vi "Transform E1, E2 using map calib xform_PN.vi"(2 "Sx, Tx, Sy, Ty":dbl[](array[numeric])=[1.0000263372329348, -5.817138285027323e-05, 0.9999727510054321, 6.062261811624134e-05], 3 "S*cos(q), S*sin(q), Tx, Ty":dbl[](array[numeric])=[1.0763223002323654, 0.0007524070719776288, -0.14779165640104555, -0.09827403757225917], 4 "E2/G2 + O2 orig":dbl[](array[numeric])=[1.8385477776704264, 1.9097301929305215, 2.0217441886705823, 2.102764185952928, 2.1689565980547436, 2.223597346902293, 2.313108622344049, 2.386560175928841, 2.4493106687615236, 2.5040748520274185, 2.5540239094260055], 5 "E1/G1 + O1 orig":dbl[](array[numeric])=[1.8159023665858196, 1.884909478785341, 2.0019297168656713, 2.086321368481948, 2.153544842540943, 2.2091798744386204, 2.299969711011518, 2.3739532300327273, 2.436788143576289, 2.4919329317716272, 2.5414088647043536]) -> (0 "E2/G2 + O2 xformed":dbl[](array[numeric])=[1.8819715743991605, 1.958636627664691, 2.0792845484484253, 2.1665492972222093, 2.2378423031751806, 2.2966936161698364, 2.3931022818543477, 2.472213336931841, 2.539798527472872, 2.598782323211661, 2.65257936765186], 1 "E1/G1 + O1 xformed":dbl[](array[numeric])=[1.8053105952325403, 1.8795328855731468, 2.005403412269025, 2.0961774595124005, 2.1684836843979456, 2.22832537384071, 2.3259797225395, 2.4055566642245805, 2.473141848949985, 2.5324557713908873, 2.585671640828993])   [LabVIEW 2010]
uses:
  <vilib>/Analysis/Matrix/Numeric/Conversions/Array To Matrix - RA2.vi
  <vilib>/Analysis/baseanly.llb/A x Vector.vi
  <vilib>/Analysis/Matrix/NI_Matrix.lvlib
  <vilib>/Analysis/NI_AALBase.lvlib
panel:
  out "E1, E2 corrected and un-corrected against calib.":cluster{dbl[], dbl[]}[](graph)=[{[1.8159023665858196, 1.884909478785341, 2.0019297168656713, 2.086321368481948, 2.153544842540943, 2.2091798744386204, 2.299969711011518, 2.3739532300327273, 2.436788143576289, 2.4919329317716272, 2.5414088647043536], [1.8385477776704264, 1.9097301929305215, 2.0217441886705823, 2.102764185952928, 2.1689565980547436, 2.223597346902293, 2.313108622344049, 2.386560175928841, 2.4493106687615236, 2.5040748520274185, 2.5540239094260055]}, {[1.8053105952325403, 1.8795328855731468, 2.005403412269025, 2.0961774595124005, 2.1684836843979456, 2.22832537384071, 2.3259797225395, 2.4055566642245805, 2.473141848949985, 2.5324557713908873, 2.585671640828993], [1.8819715743991605, 1.958636627664691, 2.0792845484484253, 2.1665492972222093, 2.2378423031751806, 2.2966936161698364, 2.3931022818543477, 2.472213336931841, 2.539798527472872, 2.598782323211661, 2.65257936765186]}]
  # "Paul Nathan 16/02/10"
  # "Transformation equations given below"
  # "First apply uniform scaling with rotation and translation:"
  # "then apply independent scaling with translation onto the points mapped with the above transformation (as a final correction, typically small)"
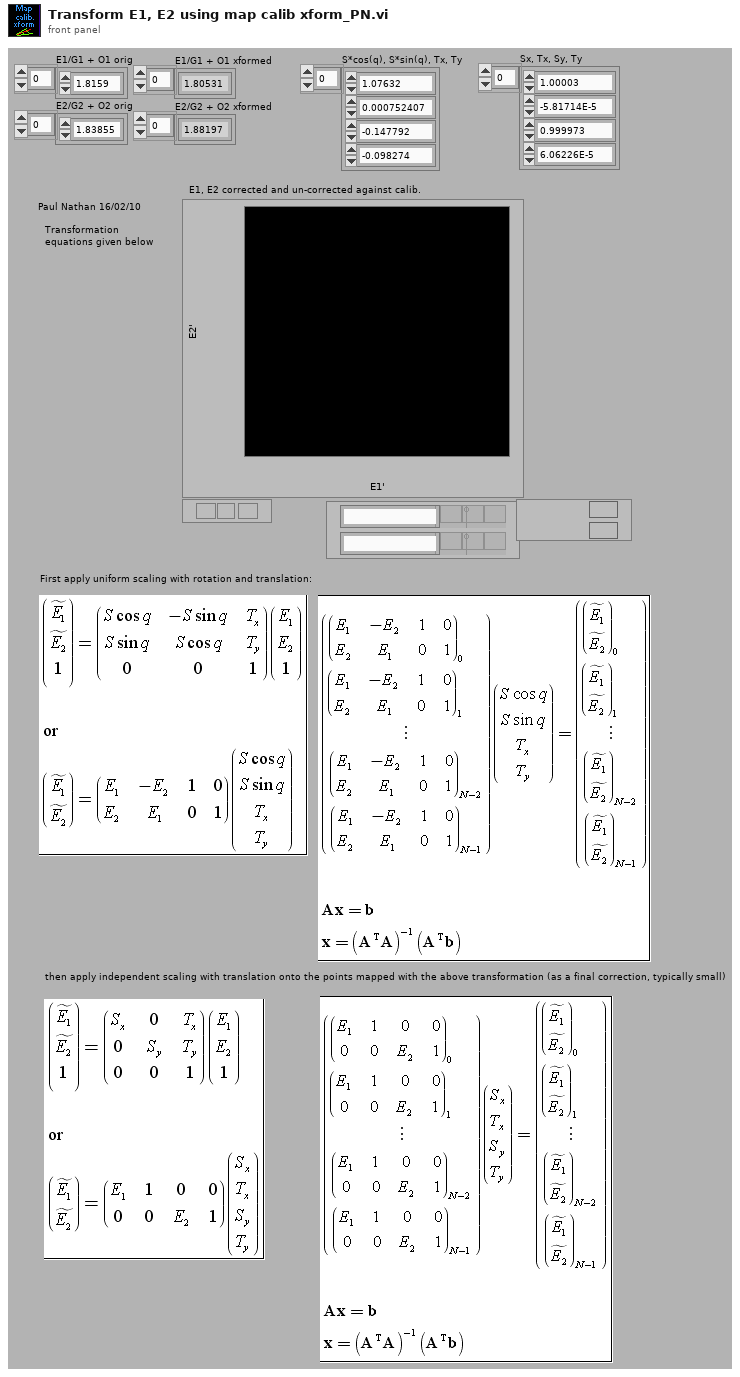
[diagram p1: front panel]
types:
  T1 = cluster{"E1/G1 + O1 orig":dbl[], "E2/G2 + O2 orig":dbl[]}
  T2 = typedef "NI_Matrix.lvlib/RealMatrix.ctl" = dbl[][]
  T3 = cluster{"E1/G1 + O1 orig":dbl[], "E2/G2 + O2 orig":dbl[]}[]
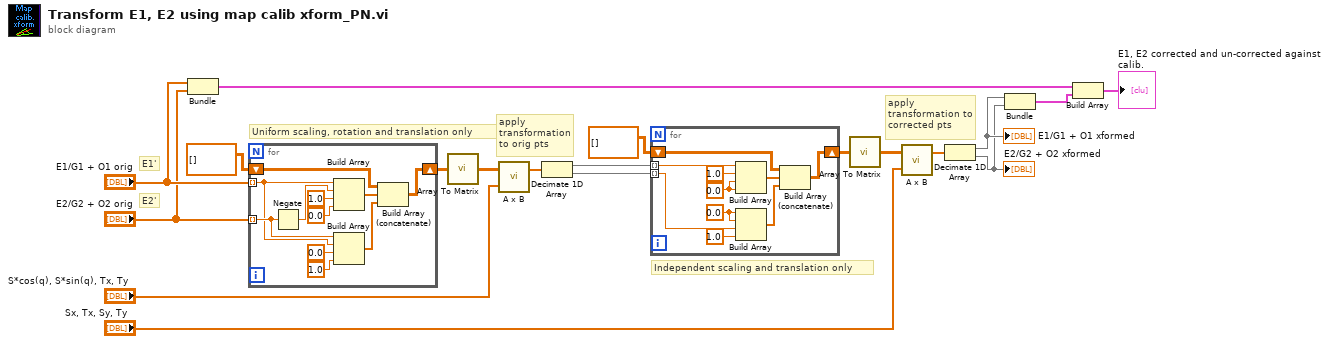
[diagram p0: block diagram]
diagram:
  # "apply transformation to corrected pts"
  # "apply transformation to orig pts"
  # "Independent scaling and translation only"
  # "Uniform scaling, rotation and translation only"
  # "E2'"
  # "E1'"
  n1 = Bundle("E1/G1 + O1 orig"="E1/G1 + O1 orig", "E2/G2 + O2 orig"="E2/G2 + O2 orig") -> (w6:T1)  [unwired: 1 out]
  n2 = for {
    tunnel: "E1/G1 + O1 orig" -> [w24] mode=indexing
    tunnel: "E2/G2 + O2 orig" -> [w25] mode=indexing
    shift-right: [w23] -> w16
    shift-left: dbl[][] [] -> [w22]
    n3 = Negate(x=w25) -> (-x=w30:dbl)
    n4 = Build Array(w24, w30, 1.0 ("element"), 0.0 ("element")) -> (w21:dbl[])
    n5 = Build Array(w25, w24, 0.0 ("element"), 1.0 ("element")) -> (w20:dbl[])
    n6 = Build Array (concatenate)(w22, w21, w20) -> (w23:dbl[][])
  }
  n7 = call-poly <vilib>:"Array To Matrix.vi"("Real 2D Array"=w16) -> ("Real Matrix"=w15:T2)
  n8 = call-poly <vilib>:"A x B.vi"("Vector"="S*cos(q), S*sin(q), Tx, Ty", "A"=w15) -> ("A x Vector"=w14:dbl[])  [unwired: 1 out]
  n9 = Decimate 1D Array(w14) -> (w12:dbl[], w13:dbl[])
  n10 = for {
    tunnel: w12 -> [w39] mode=indexing
    tunnel: w13 -> [w33] mode=indexing
    shift-right: [w38] -> w18
    shift-left: dbl[][] [] -> [w37]
    w31 = 0.0 ("element")
    w32 = 0.0 ("element")
    n11 = Build Array(w39, 1.0 ("element"), w32, w32) -> (w36:dbl[])
    n12 = Build Array(w31, w31, w33, 1.0 ("element")) -> (w35:dbl[])
    n13 = Build Array (concatenate)(w37, w36, w35) -> (w38:dbl[][])
  }
  n14 = call-poly <vilib>:"Array To Matrix.vi"("Real 2D Array"=w18) -> ("Real Matrix"=w11:T2)
  n15 = call-poly <vilib>:"A x B.vi"("Vector"="Sx, Tx, Sy, Ty", "A"=w11) -> ("A x Vector"=w9:dbl[])  [unwired: 1 out]
  n16 = Decimate 1D Array(w9) -> (w8:dbl[], w7:dbl[])
  "E1/G1 + O1 xformed" <- w8
  "E2/G2 + O2 xformed" <- w7
  n17 = Bundle(w8, w7) -> (w5:cluster{dbl[], dbl[]})  [unwired: 1 out]
  n18 = Build Array(w6, w5) -> (→"E1, E2 corrected and un-corrected against calib.":T3)
